vi "Wait for safety button.vi"(6 "Button Info":refnum<vi>, 8 "error in (no error)":errorcluster, 10 "device ID in":refnum<k1>, 11 "Calibration Cluster in":T1) -> (0 "error out":errorcluster, 2 "Refnum out":refnum<k1>, 3 "Calibration Cluster out":T1)   [LabVIEW 2014]
uses:
  Controls/Controllers Clusters/Game Pad Calibration Cluster.ctl
  <vilib>/Utility/inputDevices.llb/joystickAcquire.vi
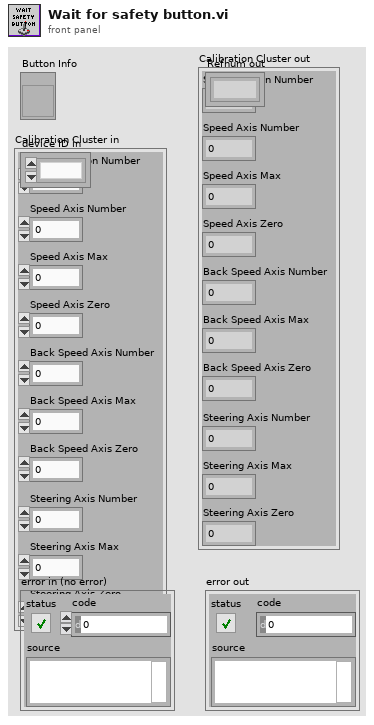
[diagram p1: front panel]
types:
  T1 = typedef "Game Pad Calibration Cluster.ctl" = cluster{"Safety Button Number":u8, "Speed Axis Number":u8, "Speed Axis Max":i32, "Speed Axis Zero":i32, "Back Speed Axis Number":u8, "Back Speed Axis Max":i32, "Back Speed Axis Zero":i32, "Steering Axis Number":u8, "Steering Axis Max":i32, "Steering Axis Zero":i32}
  T2 = cluster{"button 1":bool, "button 2":bool, "button 3":bool, "button 4":bool, "button 5":bool, "button 6":bool, "button 7":bool, "button 8":bool, "button 9":bool, "button 10":bool, "button 11":bool, "button 12":bool, "button 13":bool, "button 14":bool, "button 15":bool, "button 16":bool, "button 17":bool, "button 18":bool, "button 19":bool, "button 20":bool, "button 21":bool, "button 22":bool, "button 23":bool, "button 24":bool, "button 25":bool, "button 26":bool, "button 27":bool, "button 28":bool, "button 29":bool, "button 30":bool, "button 31":bool, "button 32":bool}
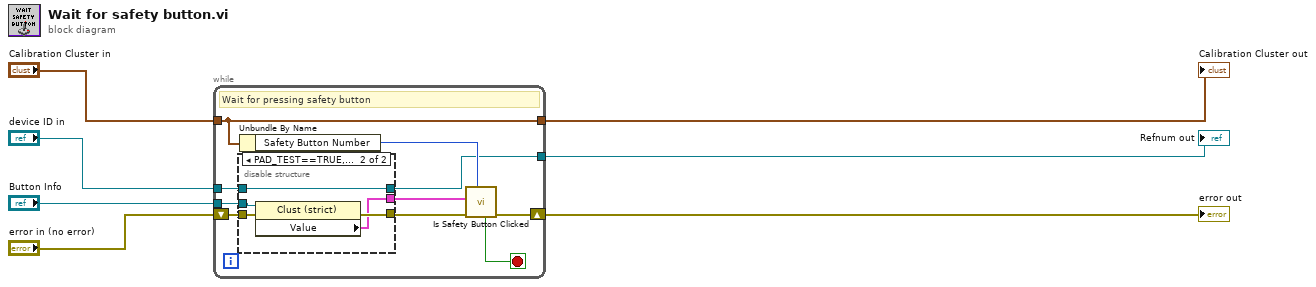
[diagram p0: block diagram]
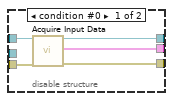
[diagram p2: hidden frame]
diagram:
  n1 = while {
    shift-right: [w12] -> w7
    shift-left: "error in (no error)" -> [w17]
    tunnel: "device ID in" -> [w16]
    tunnel: "Calibration Cluster in" -> [w9]
    tunnel: [w10] -> w5
    tunnel: [w9] -> w6
    tunnel: "Button Info" -> [w8]
    stop <- w11 stop-if-true
    # "Wait for pressing safety button"
    n2 = disable-structure shown="PAD_TEST==TRUE, Default" {
      disable-tunnel: w17 -> [w22 w26]
      disable-tunnel: w16 -> [w21 w27]
      disable-tunnel: [w20 w27] -> w10
      disable-tunnel: [w19 w23] -> w13
      disable-tunnel: [w18 w25] -> w15
      disable-tunnel: w8 -> [_ w24]
      frame condition #0 {
        n3 = call-poly <vilib>:"Acquire Input Data.vi"("device ID"=w21, "error in (no error)"=w22) -> ("device ID"=w20:refnum<k1>, "button info"=w19:T2, "error out"=w18:errorcluster)  [unwired: 13 in, 2 out]
      }
      frame condition #1 (active) {
        n4 = property on="Property Node" class="Clust (strict)"(reference=w24, error in=w26) -> (error out=w25:errorcluster, "Value"=w23:T2)  [unwired: 1 out]
      }
    }
    n5 = Unbundle By Name(w9) -> ("Safety Button Number"=w14:u8)
    n6 = call "Is Safety Button Clicked.vi"("Safety Button Number"=w14, "Error In"=w15, "Button Info"=w13) -> ("Error Out"=w12:errorcluster, "Clicked?"=w11:bool)  [unwired: 7 in]
  }
  "error out" <- w7
  "Calibration Cluster out" <- w6
  "Refnum out" <- w5
